vi "final gps synchronization with recursive.vi"() -> ()   [LabVIEW 2014]
uses:
  <vilib>/FPGAPlugInAG/cRIO-9063/niLvFpga_Open_cRIO-9063.vi
  <vilib>/rvi/interface/common/dynamic/niFpgaDynamicAddResources.vi
  <vilib>/Utility/error.llb/Error Cluster From Error Code.vi
  <vilib>/rvi/errors/niLvFpgaAdjustHostInterfaceError.vi
  <vilib>/FPGAPlugInAG/Dynamic/niLvFpga_Close_Dynamic.vi
  <vilib>/rvi/interface/nirviOpenFPGA/nirviOpenFPGA.xnode
  akhil3/FPGA Bitfiles/trailswithgps_FPGATarget_recursiveakhil_QexfQQGvF84.lvbitx
  recursive akhil.vi
  akhil3/FPGA Bitfiles/trailswithgps_FPGATarget2_recursive2_3NDbUzkOS+M.lvbitx
  <vilib>/rvi/interface/nirviReadWriteControl/nirviReadWriteControl.xnode
  <vilib>/rvi/interface/nirviCloseFPGA/nirviCloseFPGA.xnode
  NiFpgaLv.dll
  <vilib>/rvi/interface/Simulation/niFpgaSimulationCallBeginRW.vi
panel:
  out "LabVIEW time":timestamp
  out "GPS status":T1(ring)
  out "FPGA Timekeeper locked":bool
  out "offset from time reference":i32
  out "Satellites Available":u8
  out "UTC offset":i8
  out "UTC offset valid":bool
  out "Frequency 3":fxp<+/-,35,18>
  out "current frequency":fxp<+/-,35,18>
  out "PPS Timestamp (TAI ns)":u64
  out "PPS TAI Timestamp":timestamp format="%<%.9X\n%x>T"
  out "PPS UTC Timestamp":timestamp format="%<%.9X\n%x>T"
  out "antenna status":T2(ring)
  out "Latitude (°)":fxp<+/-,28,8>
  out "Longitude (°)":fxp<+/-,29,9>
  out "Altitude (m)":fxp<+/-,24,17>
  out "ROCOF 3":fxp<+/-,17,17>
  out "Theta":fxp<+/-,22,10>[](array[numeric])
  out "Magnitude":fxp<+,60,17>[](array[numeric])
  out "Current Phasor":picture
  in  "polar attributes 6":T3={"maximum"=0.0, "minimum"=0.0, "clip to min"=FALSE, "log?(F)"=FALSE, "grid color"=6710886, "plot color"=65280, "fmt and prec"={"format"=enum."Decimal", "precision"=0}, "visible section"=8} {"minimum" format="%0.2f"; "maximum" format="%0.2f"}
  out "Voltage Phasor":picture
  in  "polar attributes 7":T3={"maximum"=0.0, "minimum"=0.0, "clip to min"=FALSE, "log?(F)"=FALSE, "grid color"=6710886, "plot color"=65280, "fmt and prec"={"format"=enum."Decimal", "precision"=0}, "visible section"=8} {"minimum" format="%0.2f"; "maximum" format="%0.2f"}
  out "?":cluster{fxp<+/-,22,10>[]}[](array[cluster])
  out "?":cluster{fxp<+,60,17>[]}[](array[cluster])
  out "?":cluster{fxp<+/-,22,10>[]}[](array[cluster])
  out "?":cluster{fxp<+,60,17>[]}[](array[cluster])
  in  "Size":u16=1
  out "Waveform Chart":dynamicdata(graph)
  out "LabVIEW time 2":timestamp
  out "GPS status 2":T1(ring)
  out "FPGA Timekeeper locked 2":bool
  out "offset from time reference 2":i32
  out "Satellites Available 2":u8
  out "UTC offset 2":i8
  out "UTC offset valid 2":bool
  out "Frequency3":fxp<+/-,35,18>
  out "current frequency 2":fxp<+/-,35,18>
  out "PPS Timestamp (TAI ns) 2":u64
  out "PPS TAI Timestamp 2":timestamp format="%<%.9X\n%x>T"
  out "PPS UTC Timestamp 2":timestamp format="%<%.9X\n%x>T"
  out "antenna status 2":T2(ring)
  out "Latitude (°) 2":fxp<+/-,28,8>
  out "Longitude (°) 2":fxp<+/-,29,9>
  out "Altitude (m) 2":fxp<+/-,24,17>
  out "ROCOF 2":fxp<+/-,17,17>
  out "Theta 2":fxp<+/-,22,10>[](array[numeric])
  out "Magnitude 2":fxp<+,60,17>[](array[numeric])
  out "Current Phasor  2":picture
  in  "polar attributes 8":T3={"maximum"=0.0, "minimum"=0.0, "clip to min"=FALSE, "log?(F)"=FALSE, "grid color"=6710886, "plot color"=65280, "fmt and prec"={"format"=enum."Decimal", "precision"=0}, "visible section"=8} {"minimum" format="%0.2f"; "maximum" format="%0.2f"}
  out "Voltage Phasor  2":picture
  in  "polar attributes 9":T3={"maximum"=0.0, "minimum"=0.0, "clip to min"=FALSE, "log?(F)"=FALSE, "grid color"=6710886, "plot color"=65280, "fmt and prec"={"format"=enum."Decimal", "precision"=0}, "visible section"=8} {"minimum" format="%0.2f"; "maximum" format="%0.2f"}
  out "?":cluster{fxp<+/-,22,10>[]}[](array[cluster])
  out "?":cluster{fxp<+,60,17>[]}[](array[cluster])
  out "?":cluster{fxp<+/-,22,10>[]}[](array[cluster])
  out "?":cluster{fxp<+,60,17>[]}[](array[cluster])
  in  "Size 2":u16=1
  out "Waveform Chart 2":dynamicdata(graph)
  out "Frequency Comparision":dynamicdata(graph)
  out "Total VAR":dbl
  out "Total W":dbl
  out "Power factor":dbl
  out "Total VA":dbl
  out "Total VAR 2":dbl
  out "Total W 2":dbl
  out "Power factor 2":dbl
  out "Total VA 2":dbl
  out "Load angle 2":dbl(graph)
  out "Load angle":dbl
  out "GPS TIMESTAMP":timestamp[](array[timestamp])
  in  "Numeric":i32
  out "Frequency":fxp<+/-,35,18>[](array[numeric])
  out "ROCOF":fxp<+/-,17,17>[](array[numeric])
  out "Frequency 2":fxp<+/-,50,19>[](array[numeric])
  out "ROCOF2":fxp<+/-,26,12>[](array[numeric])
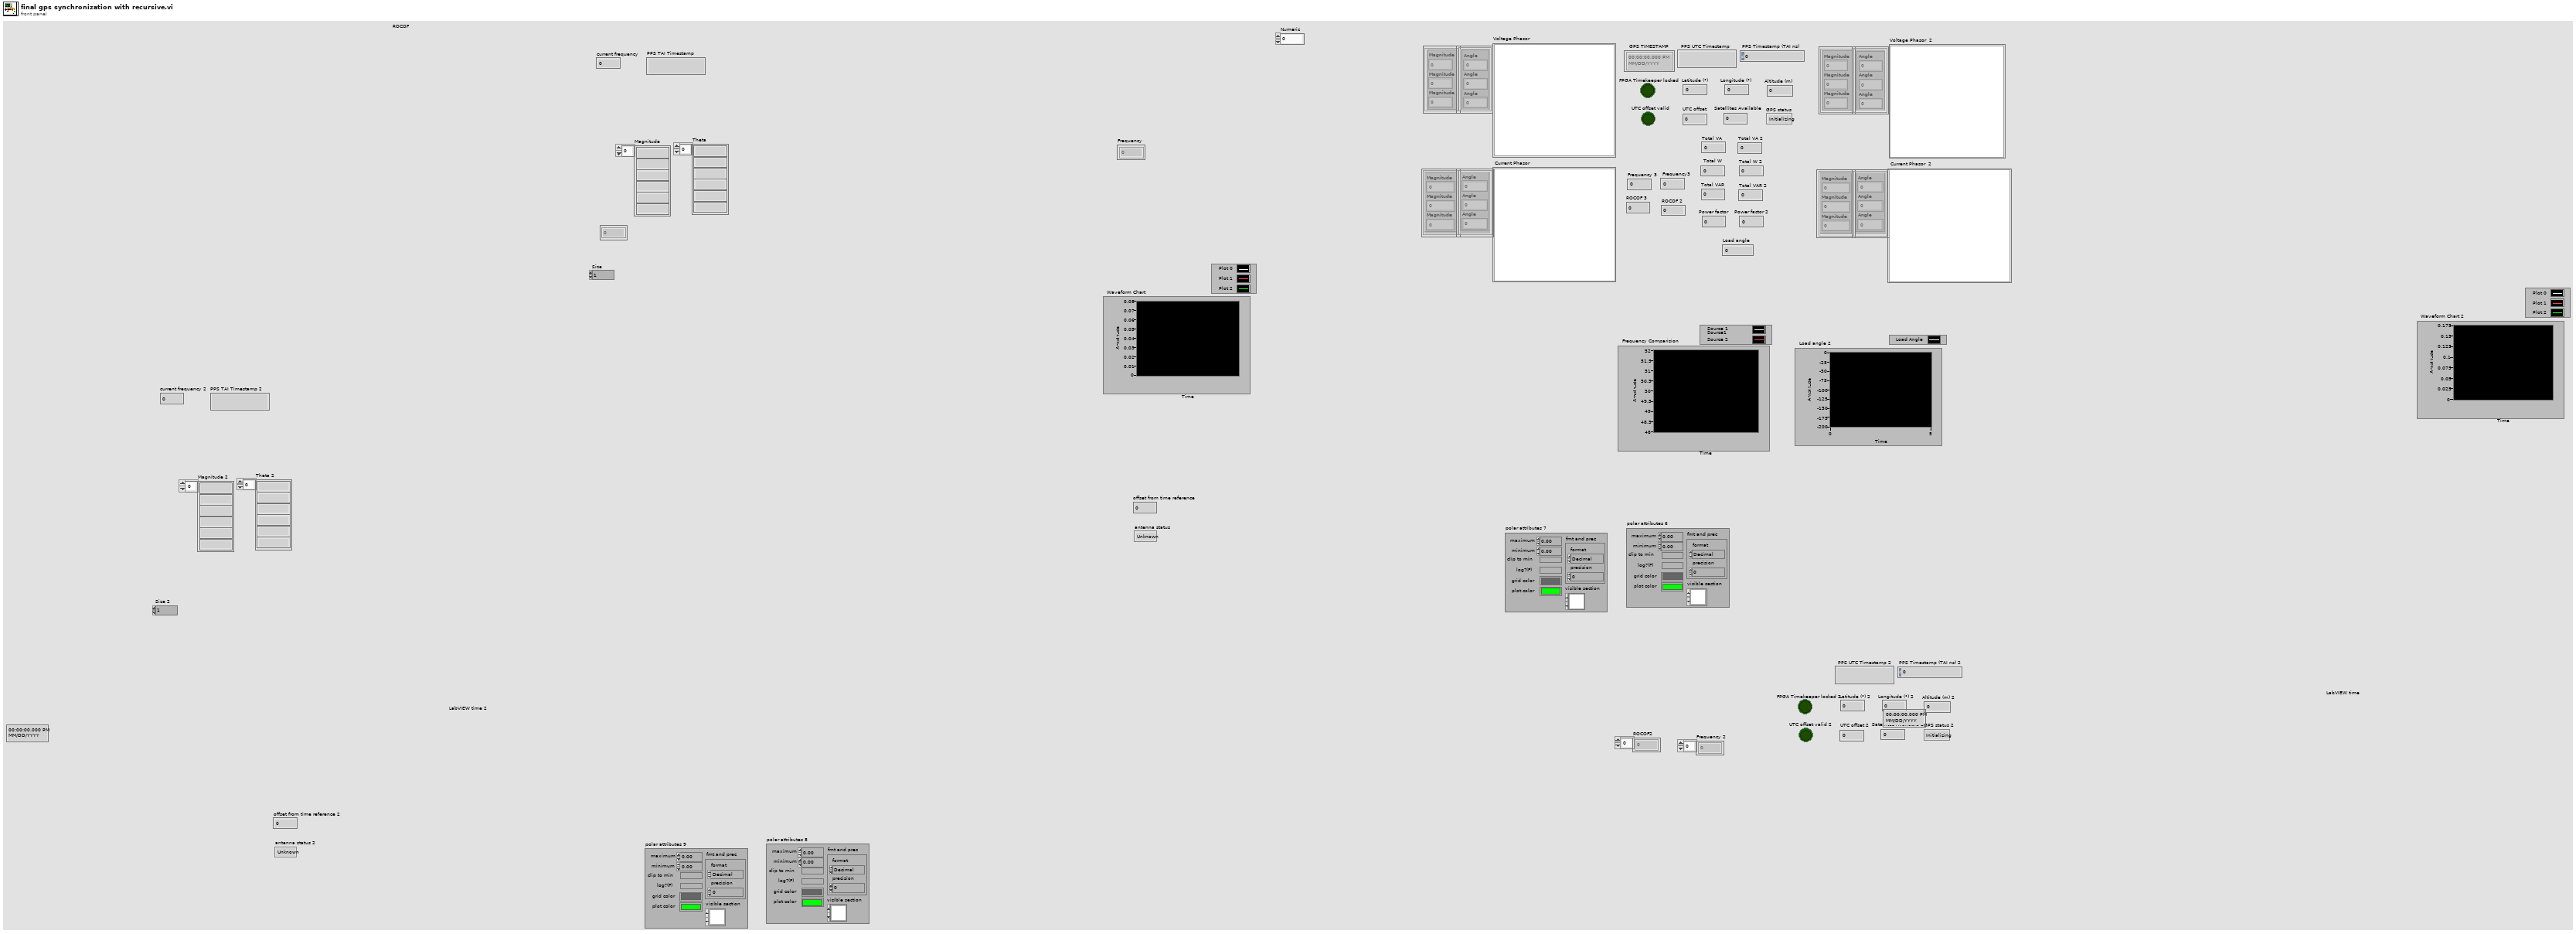
[diagram p1: front panel]
types:
  T1 = enum8{"Initializing", "Normal", "Unable to get fix"}
  T2 = enum8{"Unknown", "Normal", "Absent", "Overcurrent"}
  T3 = cluster{"maximum":dbl, "minimum":dbl, "clip to min":bool, "log?(F)":bool, "grid color":u32, "plot color":u32, "fmt and prec":cluster{"format":enum8{"Decimal", "Scientific", "Engineering", "Binary", "Octal", "Hex"}, "precision":u8}, "visible section":u16}
  T4 = cluster{"magnitude":fxp<+,60,17>, "element":fxp<+/-,61,18>}[]
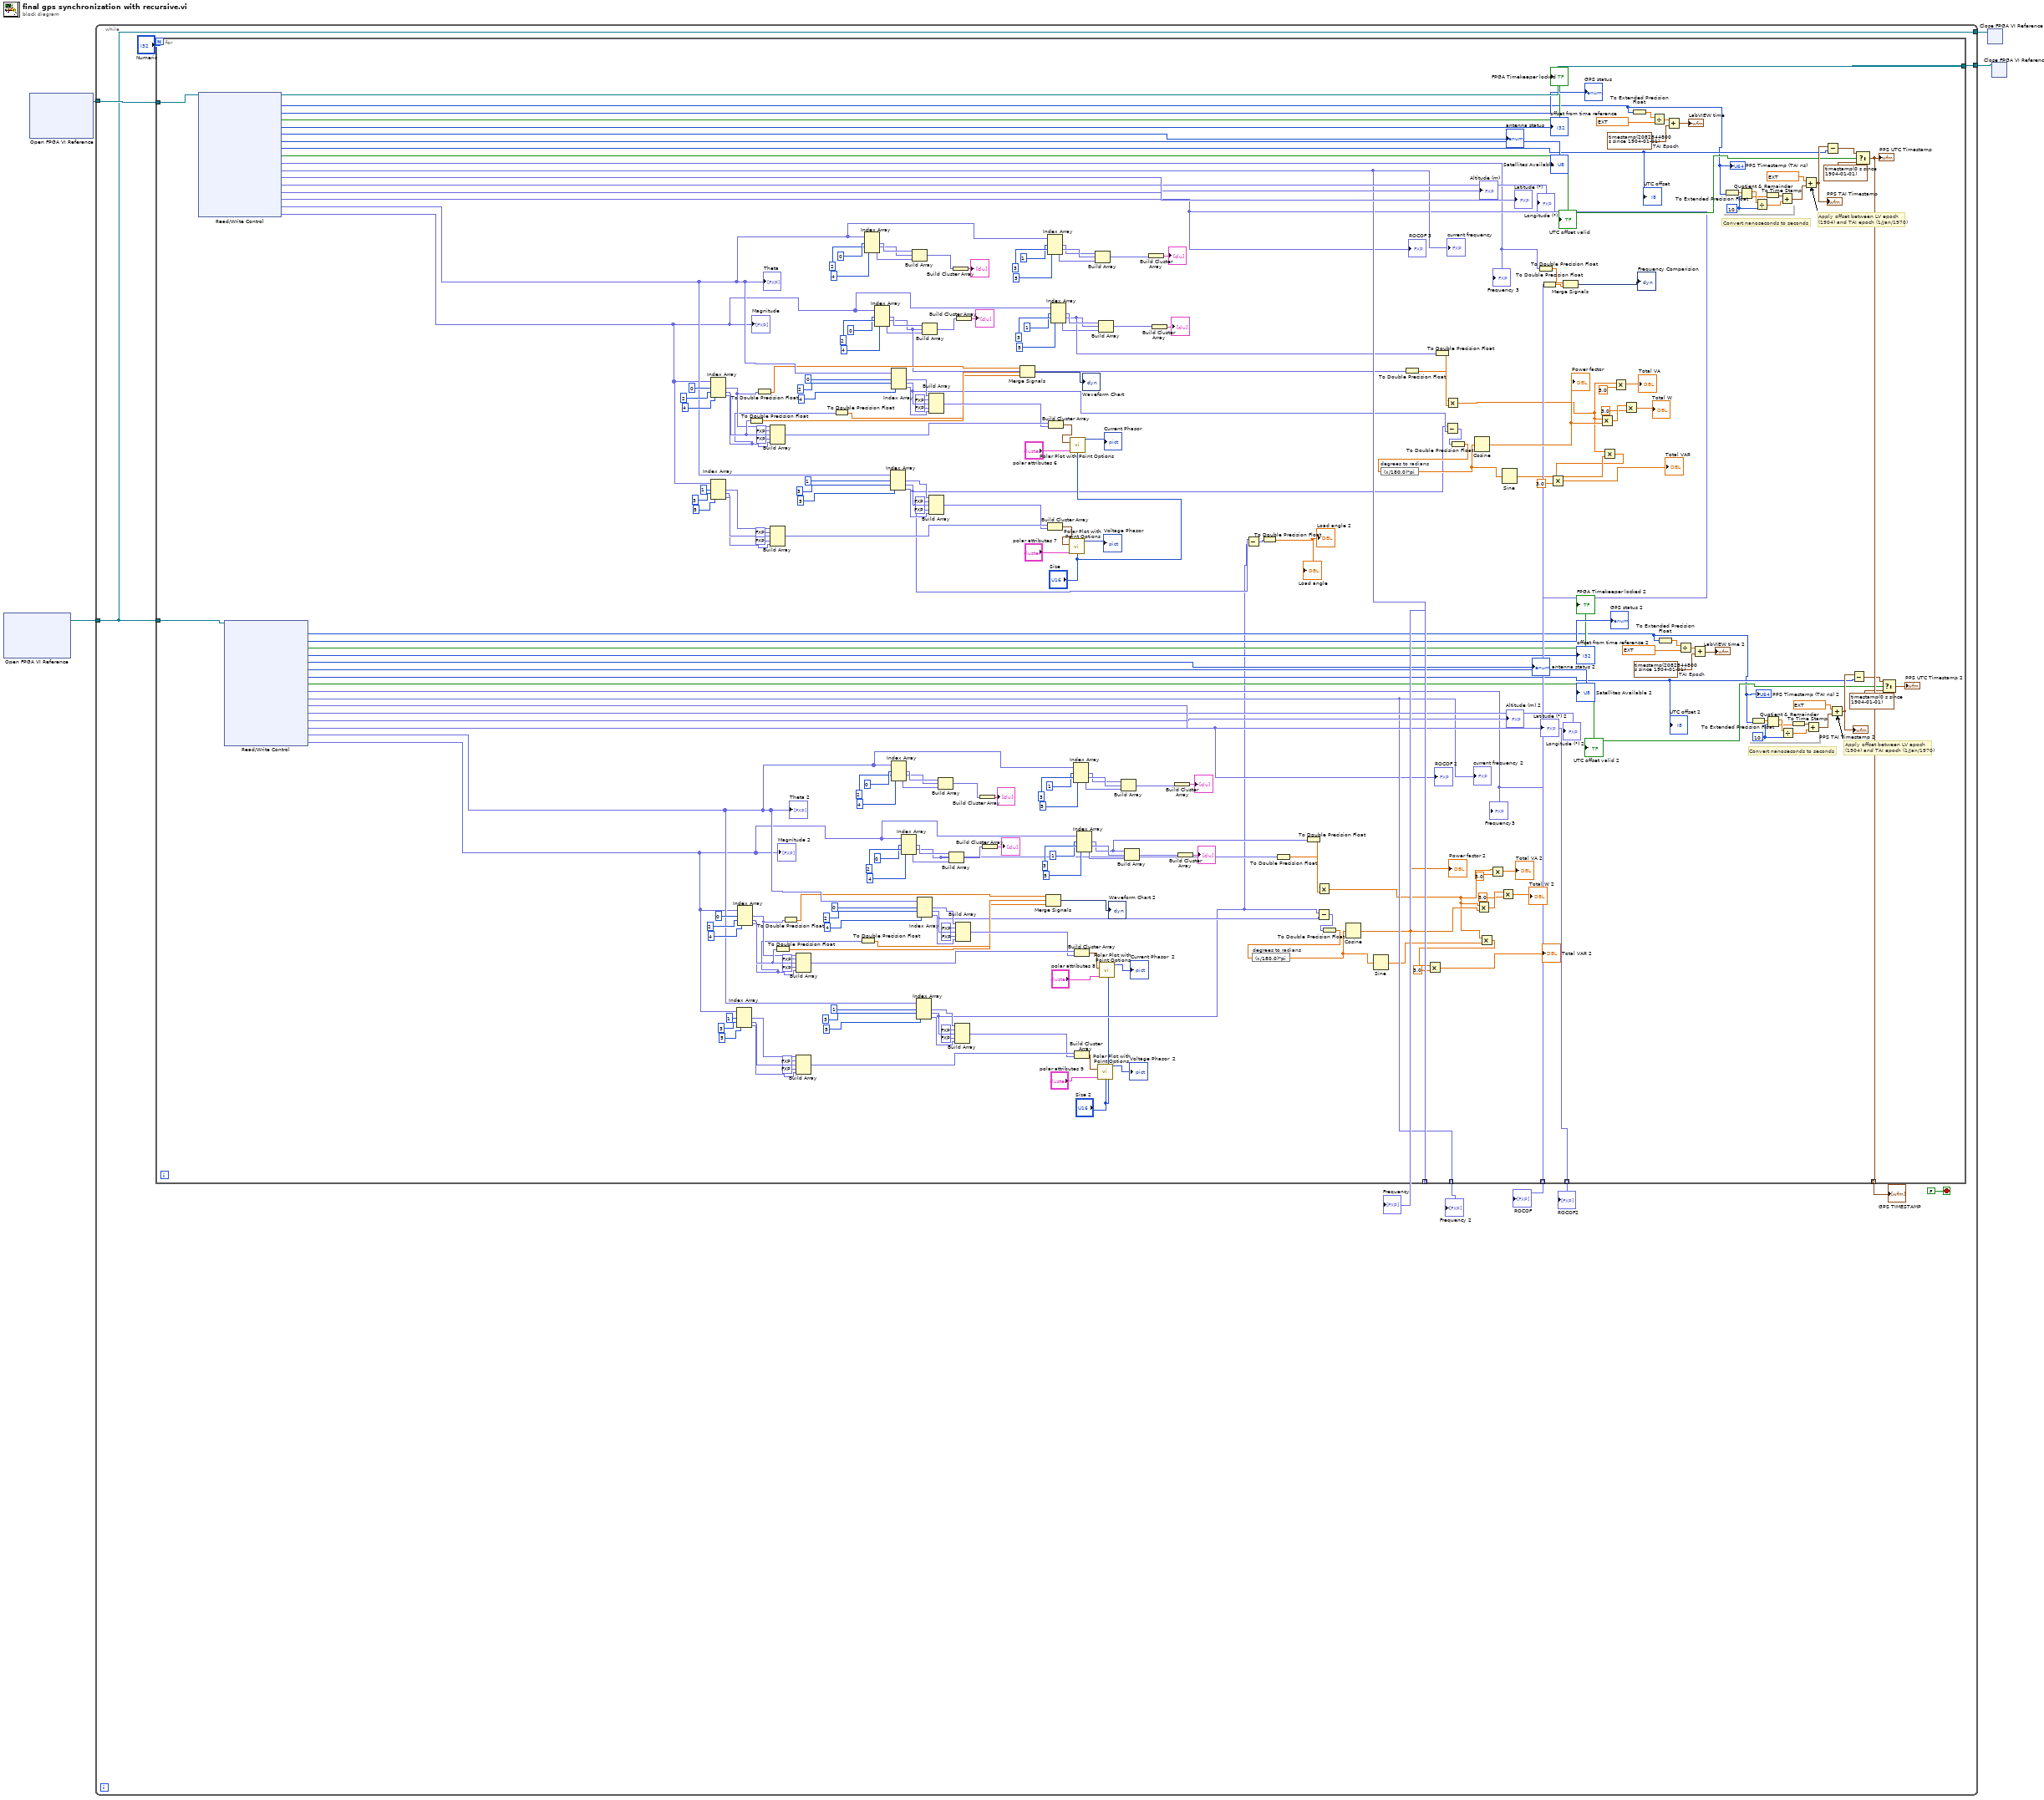
[diagram p0: block diagram]
diagram:
  n1 = xnode "Open FPGA VI Reference"() -> ("FPGA VI Reference Out"=w2:refnum<k20>)  [unwired: 2 in, 1 out]
  n2 = xnode "Open FPGA VI Reference"() -> ("FPGA VI Reference Out"=w3:refnum<k20>)  [unwired: 2 in, 1 out]
  n3 = while {
    tunnel: [w13] -> w4
    tunnel: w3 -> [w11]
    tunnel: w2 -> [w5]
    tunnel: [w5] -> w1
    stop <- FALSE stop-if-true
    n4 = for {
      N: "Numeric" -> [_]
      tunnel: w11 -> [w273]
      tunnel: [w272] -> w13
      tunnel: [w252] -> w14 mode=indexing
      tunnel: [w186] -> w9 mode=indexing
      tunnel: [w185] -> w8 mode=indexing
      tunnel: w5 -> [w79]
      tunnel: [w78] -> w7 mode=indexing
      tunnel: [w77] -> w6 mode=indexing
      w166 = u32 1000000000
      w175 = timestamp(2082844800 s since 1904-01-01)  # TAI Epoch
      w265 = u32 1000000000
      w276 = timestamp(2082844800 s since 1904-01-01)  # TAI Epoch
      # "Apply offset between LV epoch (1904) and TAI epoch (1/Jan/1970)"
      # "Convert nanoseconds to seconds"
      # "Apply offset between LV epoch (1904) and TAI epoch (1/Jan/1970)"
      # "Convert nanoseconds to seconds"
      n5 = xnode "Read/Write Control"("FPGA VI Reference In"=w273) -> ("FPGA VI Reference Out"=w272:refnum<k20>, "FPGA Timekeeper time (ns) 2"=w253:u64, "GPS status"=→"GPS status":T1, "FPGA Timekeeper locked"=→"FPGA Timekeeper locked":bool, "offset from time reference"=→"offset from time reference":i32, "antenna status"=→"antenna status":T2, "satellites available"=→"Satellites Available":u8, "UTC offset"=w255:i8, "UTC offset valid"=w256:bool, "Voltage Frequency"=w60:fxp<+/-,35,18>, "current frequency"=w186:fxp<+/-,35,18>, "Latitude (°)"=→"Latitude (°)":fxp<+/-,28,8>, "Longitude (°)"=→"Longitude (°)":fxp<+/-,29,9>, "Altitude (m)"=→"Altitude (m)":fxp<+/-,24,17>, "ROCOF"=w185:fxp<+/-,17,17>, "theta"=w203:fxp<+/-,22,10>[], "r"=w196:fxp<+,60,17>[])  [unwired: 1 in, 1 out]
      "UTC offset" <- w255
      "UTC offset valid" <- w256
      "Frequency 3" <- w60
      "current frequency" <- w186
      "PPS Timestamp (TAI ns)" <- w253
      "ROCOF 3" <- w185
      "Theta" <- w203
      "Magnitude" <- w196
      n6 = xnode "Read/Write Control"("FPGA VI Reference In"=w79) -> ("FPGA Timekeeper time (ns) 2"=w154:u64, "GPS status"=→"GPS status 2":T1, "FPGA Timekeeper locked"=→"FPGA Timekeeper locked 2":bool, "offset from time reference"=→"offset from time reference 2":i32, "antenna status"=→"antenna status 2":T2, "satellites available"=→"Satellites Available 2":u8, "UTC offset"=w156:i8, "UTC offset valid"=w157:bool, "Voltage Frequency"=w59:fxp<+/-,35,18>, "current frequency"=w78:fxp<+/-,35,18>, "Latitude (°)"=→"Latitude (°) 2":fxp<+/-,28,8>, "Longitude (°)"=→"Longitude (°) 2":fxp<+/-,29,9>, "Altitude (m)"=→"Altitude (m) 2":fxp<+/-,24,17>, "ROCOF"=w77:fxp<+/-,17,17>, "theta"=w106:fxp<+/-,22,10>[], "r"=w95:fxp<+,60,17>[])  [unwired: 1 in, 2 out]
      "UTC offset 2" <- w156
      "UTC offset valid 2" <- w157
      "Frequency3" <- w59
      "current frequency 2" <- w78
      "PPS Timestamp (TAI ns) 2" <- w154
      "ROCOF 2" <- w77
      "Theta 2" <- w106
      "Magnitude 2" <- w95
      n7 = Index Array(array=w196, index #1=1 ("index"), index #2=3 ("index"), index #3=5 ("index")) -> (element #1=w227:fxp<+,60,17>, element #2=w225:fxp<+,60,17>, element #3=w223:fxp<+,60,17>)
      n8 = Index Array(array=w196, index #1=0 ("index"), index #2=2 ("index"), index #3=4 ("index")) -> (element #1=w182:fxp<+,60,17>, element #2=w184:fxp<+,60,17>, element #3=w180:fxp<+,60,17>)
      n9 = Index Array(array=w95, index #1=1 ("index"), index #2=3 ("index"), index #3=5 ("index")) -> (element #1=w129:fxp<+,60,17>, element #2=w127:fxp<+,60,17>, element #3=w125:fxp<+,60,17>)
      n10 = Index Array(array=w95, index #1=0 ("index"), index #2=2 ("index"), index #3=4 ("index")) -> (element #1=w84:fxp<+,60,17>, element #2=w86:fxp<+,60,17>, element #3=w82:fxp<+,60,17>)
      n11 = To Double Precision Float(number=w184) -> (double precision float=w183:dbl)
      n12 = To Double Precision Float(number=w182) -> (double precision float=w181:dbl)
      n13 = Build Array(w227, fxp<+,60,17> 0.0 ("element"), w225, fxp<+,60,17> 0.0 ("element"), w223) -> (w220:fxp<+,60,17>[])
      n14 = Build Array(w182, fxp<+,60,17> 0.0 ("element"), w184, fxp<+,60,17> 0.0 ("element"), w180) -> (w238:fxp<+,60,17>[])
      n15 = To Double Precision Float(number=w86) -> (double precision float=w85:dbl)
      n16 = To Double Precision Float(number=w84) -> (double precision float=w83:dbl)
      n17 = Build Array(w129, fxp<+,60,17> 0.0 ("element"), w127, fxp<+,60,17> 0.0 ("element"), w125) -> (w120:fxp<+,60,17>[])
      n18 = Build Array(w84, fxp<+,60,17> 0.0 ("element"), w86, fxp<+,60,17> 0.0 ("element"), w82) -> (w137:fxp<+,60,17>[])
      n19 = To Double Precision Float(number=w180) -> (double precision float=w179:dbl)
      n20 = To Double Precision Float(number=w82) -> (double precision float=w81:dbl)
      n21 = Index Array(array=w203, index #1=0 ("index"), index #2=2 ("index"), index #3=4 ("index")) -> (element #1=w212:fxp<+/-,22,10>, element #2=w211:fxp<+/-,22,10>, element #3=w210:fxp<+/-,22,10>)
      n22 = Index Array(array=w196, index #1=0 ("index"), index #2=2 ("index"), index #3=4 ("index")) -> (element #1=w74:fxp<+,60,17>, element #2=w66:fxp<+,60,17>, element #3=w61:fxp<+,60,17>)
      n23 = Index Array(array=w203, index #1=1 ("index"), index #2=3 ("index"), index #3=5 ("index")) -> (element #1=w76:fxp<+/-,22,10>, element #2=w26:fxp<+/-,22,10>, element #3=w63:fxp<+/-,22,10>)
      n24 = Index Array(array=w203, index #1=0 ("index"), index #2=2 ("index"), index #3=4 ("index")) -> (element #1=w75:fxp<+/-,22,10>, element #2=w67:fxp<+/-,22,10>, element #3=w64:fxp<+/-,22,10>)
      n25 = Index Array(array=w106, index #1=0 ("index"), index #2=2 ("index"), index #3=4 ("index")) -> (element #1=w115:fxp<+/-,22,10>, element #2=w114:fxp<+/-,22,10>, element #3=w113:fxp<+/-,22,10>)
      n26 = Index Array(array=w95, index #1=0 ("index"), index #2=2 ("index"), index #3=4 ("index")) -> (element #1=w99:fxp<+,60,17>, element #2=w39:fxp<+,60,17>, element #3=w100:fxp<+,60,17>)
      n27 = Build Array(w212, w211, w210) -> (w195:fxp<+/-,22,10>[])
      n28 = Index Array(array=w106, index #1=1 ("index"), index #2=3 ("index"), index #3=5 ("index")) -> (element #1=w122:fxp<+/-,22,10>, element #2=w25:fxp<+/-,22,10>, element #3=w121:fxp<+/-,22,10>)
      n29 = Index Array(array=w106, index #1=0 ("index"), index #2=2 ("index"), index #3=4 ("index")) -> (element #1=w139:fxp<+/-,22,10>, element #2=w38:fxp<+/-,22,10>, element #3=w138:fxp<+/-,22,10>)
      n30 = Build Array(w74, w66, w61) -> (w194:fxp<+,60,17>[])
      n31 = Build Array(w76, fxp<+,60,17> 0.0 ("element"), w26, fxp<+,60,17> 0.0 ("element"), w63) -> (w219:fxp<+/-,61,18>[])
      n32 = Build Array(w75, fxp<+,60,17> 0.0 ("element"), w67, fxp<+,60,17> 0.0 ("element"), w64) -> (w237:fxp<+/-,61,18>[])
      n33 = Build Array(w115, w114, w113) -> (w94:fxp<+/-,22,10>[])
      n34 = Build Array(w99, w39, w100) -> (w93:fxp<+,60,17>[])
      n35 = Build Cluster Array(w195) -> (→"?":cluster{fxp<+/-,22,10>[]}[])
      n36 = Build Array(w122, fxp<+,60,17> 0.0 ("element"), w25, fxp<+,60,17> 0.0 ("element"), w121) -> (w119:fxp<+/-,61,18>[])
      n37 = Build Array(w139, fxp<+,60,17> 0.0 ("element"), w38, fxp<+,60,17> 0.0 ("element"), w138) -> (w136:fxp<+/-,61,18>[])
      n38 = Build Cluster Array(w194) -> (→"?":cluster{fxp<+,60,17>[]}[])
      n39 = Build Cluster Array(w94) -> (→"?":cluster{fxp<+/-,22,10>[]}[])
      n40 = Build Cluster Array(w93) -> (→"?":cluster{fxp<+,60,17>[]}[])
      n41 = Merge Signals(w181, w183, w179) -> (→"Waveform Chart":dynamicdata)
      n42 = Merge Signals(w83, w85, w81) -> (→"Waveform Chart 2":dynamicdata)
      n43 = Index Array(array=w203, index #1=1 ("index"), index #2=3 ("index"), index #3=5 ("index")) -> (element #1=w207:fxp<+/-,22,10>, element #2=w208:fxp<+/-,22,10>, element #3=w209:fxp<+/-,22,10>)
      n44 = Build Cluster Array(w220, w219) -> (w217:T4)
      n45 = Build Cluster Array(w238, w237) -> (w235:T4)
      n46 = Index Array(array=w196, index #1=1 ("index"), index #2=3 ("index"), index #3=5 ("index")) -> (element #1=w73:fxp<+,60,17>, element #2=w65:fxp<+,60,17>, element #3=w62:fxp<+,60,17>)
      n47 = call <vilib>:"Polar Plot with Point Options.vi"("data array [mag, phase (deg)]"=w217, "polar attributes"="polar attributes 7", "Size"="Size") -> ("new picture"=→"Voltage Phasor":picture)  [unwired: 12 in]
      n48 = call <vilib>:"Polar Plot with Point Options.vi"("data array [mag, phase (deg)]"=w235, "polar attributes"="polar attributes 6", "Size"="Size") -> ("new picture"=→"Current Phasor":picture)  [unwired: 12 in]
      n49 = Index Array(array=w106, index #1=1 ("index"), index #2=3 ("index"), index #3=5 ("index")) -> (element #1=w110:fxp<+/-,22,10>, element #2=w111:fxp<+/-,22,10>, element #3=w112:fxp<+/-,22,10>)
      n50 = Build Cluster Array(w120, w119) -> (w21:T4)
      n51 = Build Cluster Array(w137, w136) -> (w18:T4)
      n52 = Index Array(array=w95, index #1=1 ("index"), index #2=3 ("index"), index #3=5 ("index")) -> (element #1=w40:fxp<+,60,17>, element #2=w104:fxp<+,60,17>, element #3=w105:fxp<+,60,17>)
      n53 = Build Array(w207, w208, w209) -> (w191:fxp<+/-,22,10>[])
      n54 = call <vilib>:"Polar Plot with Point Options.vi"("data array [mag, phase (deg)]"=w21, "polar attributes"="polar attributes 9", "Size"="Size 2") -> ("new picture"=→"Voltage Phasor  2":picture)  [unwired: 12 in]
      n55 = Build Array(w73, w65, w62) -> (w190:fxp<+,60,17>[])
      n56 = call <vilib>:"Polar Plot with Point Options.vi"("data array [mag, phase (deg)]"=w18, "polar attributes"="polar attributes 8", "Size"="Size 2") -> ("new picture"=→"Current Phasor  2":picture)  [unwired: 12 in]
      n57 = Build Array(w110, w111, w112) -> (w90:fxp<+/-,22,10>[])
      n58 = Build Array(w40, w104, w105) -> (w89:fxp<+,60,17>[])
      n59 = Build Cluster Array(w191) -> (→"?":cluster{fxp<+/-,22,10>[]}[])
      n60 = Build Cluster Array(w190) -> (→"?":cluster{fxp<+,60,17>[]}[])
      n61 = Build Cluster Array(w90) -> (→"?":cluster{fxp<+/-,22,10>[]}[])
      n62 = Build Cluster Array(w89) -> (→"?":cluster{fxp<+,60,17>[]}[])
      n63 = Subtract(x=w26, y=w25) -> (x-y=w24:fxp<+/-,23,11>)
      n64 = To Double Precision Float(number=w24) -> (double precision float=→"Load angle 2" →"Load angle":dbl)
      n65 = To Double Precision Float(number=w39) -> (double precision float=w43:dbl)
      n66 = To Double Precision Float(number=w40) -> (double precision float=w44:dbl)
      n67 = Subtract(x=w25, y=w38) -> (x-y=w45:fxp<+/-,23,11>)
      n68 = Multiply(x=w43, y=w44) -> (x*y=w27:dbl)
      n69 = To Double Precision Float(number=w45) -> (double precision float=w41:dbl)
      n70 = expression code="(x/180.0)*pi" "degrees to radians"(w41) -> (w42:dbl)
      n71 = Cosine(x=w42) -> (cos(x)=w28:dbl)
      "Power factor 2" <- w28
      n72 = Sine(x=w42) -> (sin(x)=w30:dbl)
      n73 = To Double Precision Float(number=w66) -> (double precision float=w69:dbl)
      n74 = To Double Precision Float(number=w65) -> (double precision float=w70:dbl)
      n75 = Subtract(x=w26, y=w67) -> (x-y=w72:fxp<+/-,23,11>)
      n76 = Multiply(x=w69, y=w70) -> (x*y=w48:dbl)
      n77 = To Double Precision Float(number=w72) -> (double precision float=w68:dbl)
      n78 = expression code="(x/180.0)*pi" "degrees to radians"(w68) -> (w56:dbl)
      n79 = Cosine(x=w56) -> (cos(x)=w71:dbl)
      "Power factor" <- w71
      n80 = Multiply(x=w27, y=w28) -> (x*y=w36:dbl)
      n81 = Multiply(x=w27, y=w30) -> (x*y=w29:dbl)
      n82 = Multiply(x=w29, y=3.0) -> (x*y=→"Total VAR 2":dbl)
      n83 = Multiply(x=w27, y=3.0) -> (x*y=→"Total VA 2":dbl)
      n84 = Multiply(x=w36, y=3.0) -> (x*y=→"Total W 2":dbl)
      n85 = Sine(x=w56) -> (sin(x)=w55:dbl)
      n86 = To Double Precision Float(number=w60) -> (double precision float=w23:dbl)
      n87 = To Double Precision Float(number=w59) -> (double precision float=w58:dbl)
      n88 = Merge Signals(w23, w58) -> (→"Frequency Comparision":dynamicdata)
      n89 = Multiply(x=w48, y=w71) -> (x*y=w51:dbl)
      n90 = Multiply(x=w48, y=w55) -> (x*y=w54:dbl)
      n91 = Multiply(x=w54, y=3.0) -> (x*y=→"Total VAR":dbl)
      n92 = Multiply(x=w48, y=3.0) -> (x*y=→"Total VA":dbl)
      n93 = Multiply(x=w51, y=3.0) -> (x*y=→"Total W":dbl)
      n94 = To Extended Precision Float(1:w253) -> (0:w274:ext)
      n95 = Divide(x=w274, y=ext 1000000000.0) -> (x/y=w277:ext)
      n96 = To Extended Precision Float(1:w154) -> (0:w173:ext)
      n97 = Add(x=w277, y=w276) -> (x+y=→"LabVIEW time":timestamp)
      n98 = Divide(x=w173, y=ext 1000000000.0) -> (x/y=w176:ext)
      n99 = Add(x=w176, y=w175) -> (x+y=→"LabVIEW time 2":timestamp)
      n100 = To Extended Precision Float(1:w253) -> (0:w267:ext)
      n101 = Quotient & Remainder(x=w267, y=w265) -> (x-y*floor(x/y)=w266:ext, floor(x/y)=w264:ext)
      n102 = To Extended Precision Float(1:w154) -> (0:w168:ext)
      n103 = Divide(x=w266, y=w265) -> (x/y=w262:ext)
      n104 = To Time Stamp(1:w264) -> (0:w263:timestamp)
      n105 = Quotient & Remainder(x=w168, y=w166) -> (x-y*floor(x/y)=w167:ext, floor(x/y)=w165:ext)
      n106 = Add(x=w263, y=w262) -> (x+y=w261:timestamp)
      n107 = Divide(x=w167, y=w166) -> (x/y=w163:ext)
      n108 = To Time Stamp(1:w165) -> (0:w164:timestamp)
      n109 = Add(x=ext 2082844800.0, y=w261) -> (x+y=w259:timestamp)
      "PPS TAI Timestamp" <- w259
      n110 = Add(x=w164, y=w163) -> (x+y=w162:timestamp)
      n111 = Subtract(x=w259, y=w255) -> (x-y=w258:timestamp)
      n112 = Add(x=ext 2082844800.0, y=w162) -> (x+y=w160:timestamp)
      "PPS TAI Timestamp 2" <- w160
      n113 = Subtract(x=w160, y=w156) -> (x-y=w159:timestamp)
      n114 = Select(t=w258, s=w256, f=timestamp(0 s since 1904-01-01)) -> (s? t:f=w252:timestamp)
      "PPS UTC Timestamp" <- w252
      n115 = Select(t=w159, s=w157, f=timestamp(0 s since 1904-01-01)) -> (s? t:f=→"PPS UTC Timestamp 2":timestamp)
    }
    "GPS TIMESTAMP" <- w14
    "Frequency" <- w9
    "ROCOF" <- w8
    "Frequency 2" <- w7
    "ROCOF2" <- w6
  }
  n116 = xnode "Close FPGA VI Reference"("FPGA VI Reference In"=w1) -> ()  [unwired: 1 in, 1 out]
  n117 = xnode "Close FPGA VI Reference"("FPGA VI Reference In"=w4) -> ()  [unwired: 1 in, 1 out]
